vi "FGA NL Find Node.vi"(4 "Node ID":u8) -> (0 "Record Exists?":bool, 1 "NodeRec":T1={"Node Id"=1, "ComponentSeq"=[{"Component Id"=1, "Instance Id"=0, "ServiceSeq"=[{"ServiceURI"="Service", "MajorVerNum"=1, "MinorVerNum"=1}]}]}, 2 "Node Index":i32)   [LabVIEW 2009]
uses:
  NodeRec.ctl
  ComponentRec.ctl
  ServiceRec.ctl
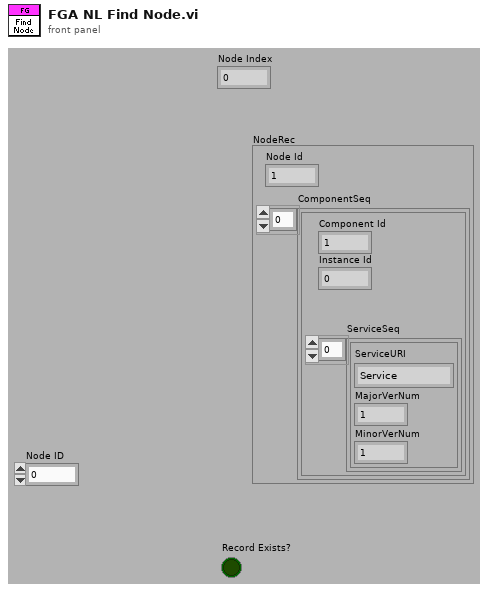
[diagram p1: front panel]
types:
  T1 = typedef "NodeRec.ctl" = cluster{"Node Id":u8, "ComponentSeq":T2[]}
  T2 = typedef "ComponentRec.ctl" = cluster{"Component Id":u8, "Instance Id":u8, "ServiceSeq":T3[]}
  T3 = typedef "ServiceRec.ctl" = cluster{"ServiceURI":string, "MajorVerNum":u8, "MinorVerNum":u8}
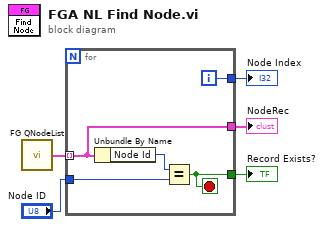
[diagram p0: block diagram]
diagram:
  n1 = call "FG QNodeList.vi"() -> ("NodeList out"=w3:T1[])  [unwired: 2 in]
  n2 = for {
    tunnel: w3 -> [w10] mode=indexing
    tunnel: "Node ID" -> [w8]
    tunnel: [w10] -> w2
    tunnel: [w7] -> w4
    tunnel: [w6] -> w1
    i -> [w6]
    stop <- w7 stop-if-true
    n3 = Unbundle By Name(w10) -> ("Node Id"=w9:u8)
    n4 = Equal?(x=w9, y=w8) -> (x = y?=w7:bool)
  }
  "Record Exists?" <- w4
  "NodeRec" <- w2
  "Node Index" <- w1
